vi "practica7MIMO.vi"() -> ()   [LabVIEW 2016]
uses:
  <vilib>/Math Plots/3D Math Plots/3D Mesh/3D Mesh XCtrl/3D Mesh.xctl
  <vilib>/addons/Fuzzy Logic/FL Fuzzy Controller (MIMO).vi
  <vilib>/Math Plots/3D Math Plots/3D Mesh/3D Mesh Datatype/Public/Plot Helper (Matrix).vi
  <vilib>/addons/Fuzzy Logic/NI_Fuzzy_Logic_API.lvlib
  <vilib>/Math Plots/3D Math Plots/3D Mesh/3D Mesh Datatype/3D Mesh Datatype.lvclass
panel:
  out "Waveform Chart 2":dbl[][](graph)
  out "Waveform Chart":dbl[][](graph)
  out "3D Mesh 2":refnum<class "3D Plot Datatype.lvclass">[](xcontrol)
  out "3D Mesh":refnum<class "3D Plot Datatype.lvclass">[](xcontrol)
  out "Motor Derecha":dbl(slide) scale=-100.0..100.0
  out "Motor Izquierda":dbl(slide) scale=-100.0..100.0
  in  "file path":path
  in  "stop":bool
  in  "Reset":bool
  out "Plano de trabajo":picture
  out "Angulo":dbl
  out "Distancia":dbl
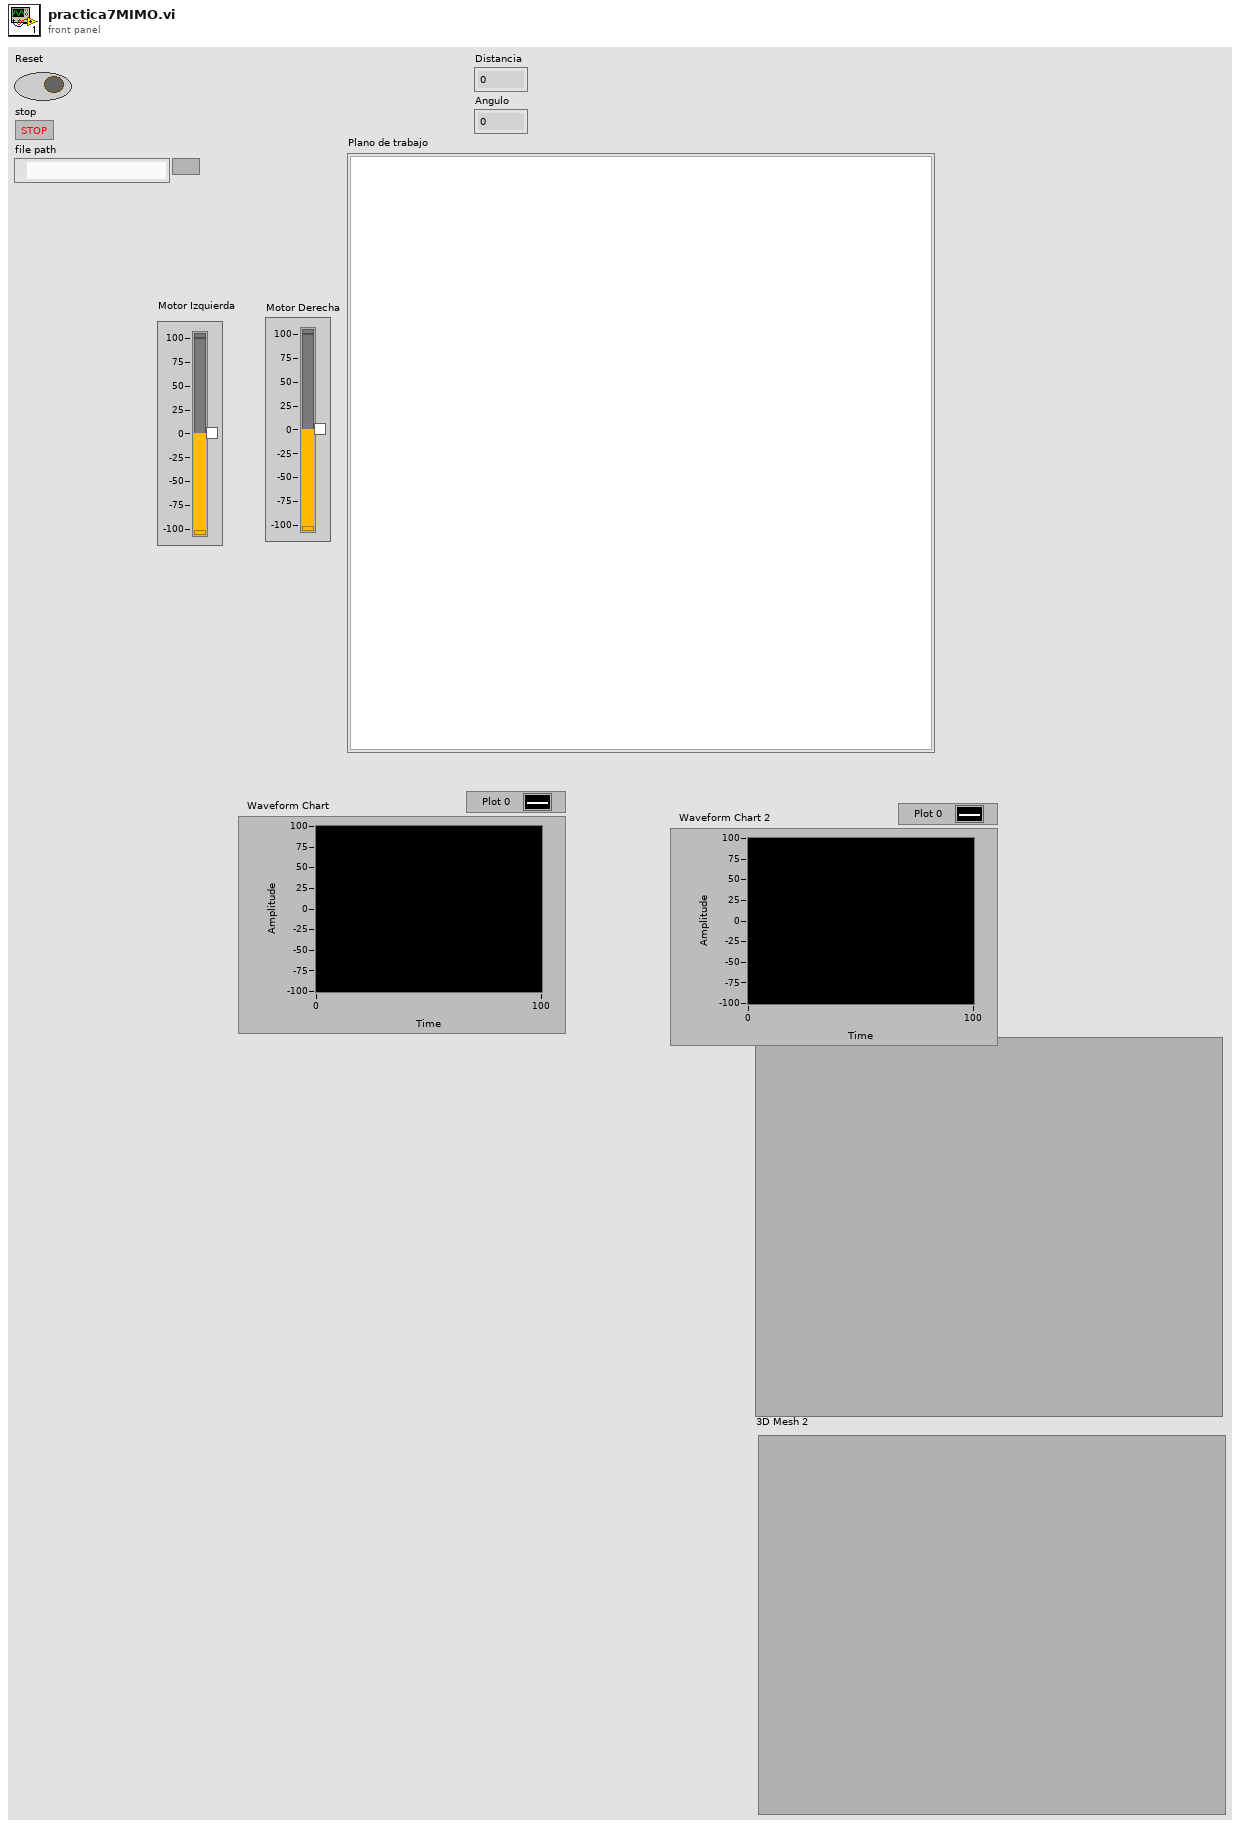
[diagram p1: front panel]
types:
  T1 = typedef "NI_Fuzzy_Logic_API.lvlib/FL System.ctl" = cluster{"input variables":T2[], "output variables":T2[], "rules":T5[], "defuzzification method":T11, "description":string, "user MF interpolating polynomials":T12[]}
  T2 = typedef "NI_Fuzzy_Logic_API.lvlib/FL Variable.ctl" = cluster{"name":string, "range":dbl[], "MFs":T3[]}
  T3 = typedef "NI_Fuzzy_Logic_API.lvlib/FL Membership Function.ctl" = cluster{"name":string, "shape":T4, "points":dbl[], "color":u32, "user-defined shape index":i32}
  T4 = typedef "NI_Fuzzy_Logic_API.lvlib/FL Membership Function Shape.ctl" = u16
  T5 = typedef "NI_Fuzzy_Logic_API.lvlib/FL Rule.ctl" = cluster{"antecedents":T6[], "antecedent connective":T8, "consequents":T9[], "consequent implication":T10, "degree of support":dbl}
  T6 = typedef "NI_Fuzzy_Logic_API.lvlib/FL Antecedent.ctl" = cluster{"Var Index":i32, "MF Index":i32, "Cond":T7}
  T7 = typedef "NI_Fuzzy_Logic_API.lvlib/FL Modifier.ctl" = u16
  T8 = typedef "NI_Fuzzy_Logic_API.lvlib/FL Antecedent Connective.ctl" = u16
  T9 = typedef "NI_Fuzzy_Logic_API.lvlib/FL Consequent.ctl" = cluster{"Var Index":i32, "MF Index":i32, "Cond":T7}
  T10 = typedef "NI_Fuzzy_Logic_API.lvlib/FL Consequent Implication.ctl" = u16
  T11 = typedef "NI_Fuzzy_Logic_API.lvlib/FL Defuzzification.ctl" = u16
  T12 = typedef "NI_Fuzzy_Logic_API.lvlib/FL Interpolating polynomials.ctl" = cluster{"X":dbl[], "Y":dbl[], "Y(x) coeff":dbl[][], "X(y) coeff":dbl[][], "Area(y) coeff":dbl[][], "coa_x(y) coeff":dbl[][]}
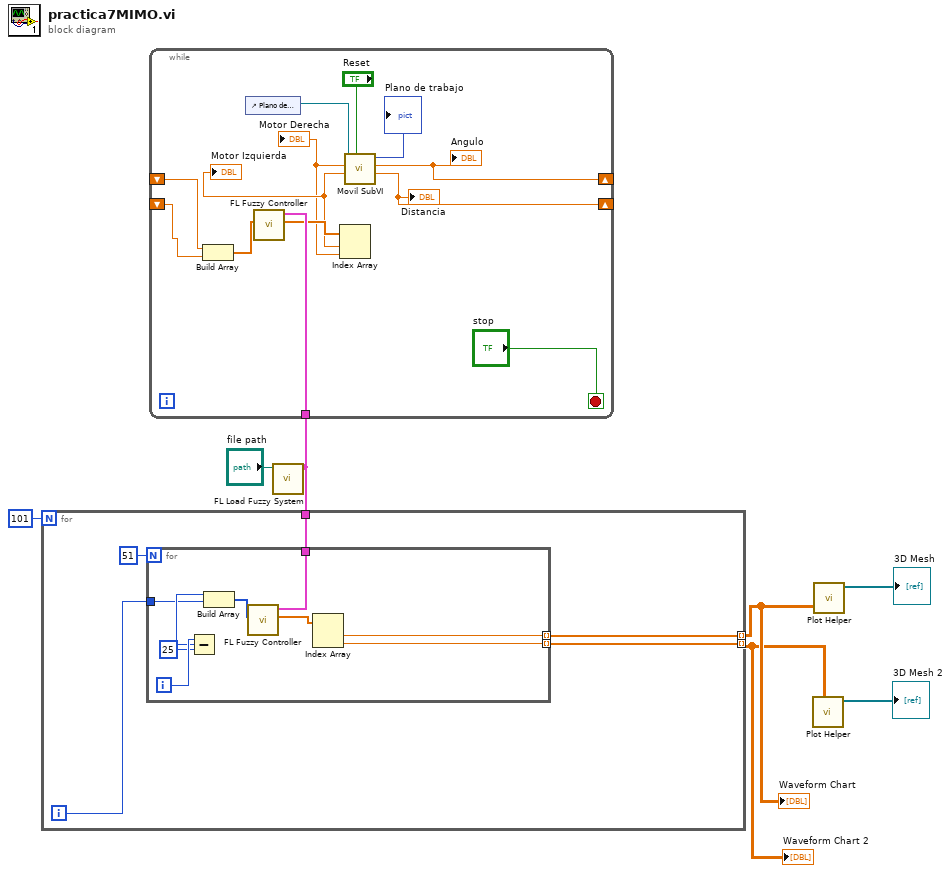
[diagram p0: block diagram]
diagram:
  n1 = call <vilib>:"FL Load Fuzzy System.vi"("file path"="file path") -> ("fuzzy system out"=w5:T1)  [unwired: 9 in, 1 out]
  n2 = for {
    N: 101 -> [_]
    tunnel: [w12] -> w2 mode=indexing
    tunnel: [w11] -> w1 mode=indexing
    tunnel: w5 -> [w8]
    i -> [w9]
    n3 = for {
      N: 51 -> [_]
      tunnel: [w20] -> w12 mode=indexing
      tunnel: [w19] -> w11 mode=indexing
      tunnel: w9 -> [w15]
      tunnel: w8 -> [w13]
      i -> [w18]
      n4 = Subtract(x=w18, y=25) -> (x-y=w16:i32)
      n5 = Build Array(w16, w15) -> (w14:i32[])
      n6 = call-poly <vilib>:"FL Fuzzy Controller.vi"("input values"=w14, "fuzzy system in"=w13) -> ("output values"=w21:dbl[])  [unwired: 5 in, 4 out]
      n7 = Index Array(array=w21) -> (element #1=w20:dbl, element #2=w19:dbl)  [unwired: 2 in]
    }
  }
  "Waveform Chart" <- w2
  "Waveform Chart 2" <- w1
  n8 = while {
    tunnel: w5 -> [w30]
    shift-right: [w28] -> _
    shift-left: _ -> [w25]
    shift-right: [w27] -> _
    shift-left: _ -> [w26]
    stop <- "stop" stop-if-true
    n9 = Build Array(w25, w26) -> (w24:dbl[])
    n10 = control-ref of="Plano de trabajo"() -> (w33:refnum<vi>)
    n11 = call-poly <vilib>:"FL Fuzzy Controller.vi"("input values"=w24, "fuzzy system in"=w30) -> ("output values"=w29:dbl[])  [unwired: 5 in, 4 out]
    n12 = Index Array(array=w29) -> (element #1=w23:dbl, element #2=w22:dbl)  [unwired: 2 in]
    "Motor Izquierda" <- w23
    "Motor Derecha" <- w22
    n13 = call "Movil SubVI.vi"("Reset"="Reset", "Motor Izquierda"=w23, "Motor Derecha"=w22, "Ref Plano"=w33) -> ("Distancia"=w27:dbl, "Angulo"=w28:dbl, "Plano de trabajo"=→"Plano de trabajo":picture)  [unwired: 3 in, 2 out]
    "Distancia" <- w27
    "Angulo" <- w28
  }
  n14 = call-poly <vilib>:"Plot Helper.vi"("z matrix"=w1) -> ("3D Plot lvclass Array out"=→"3D Mesh 2":refnum<class "3D Plot Datatype.lvclass">[])  [unwired: 5 in, 5 out]
  n15 = call-poly <vilib>:"Plot Helper.vi"("z matrix"=w2) -> ("3D Plot lvclass Array out"=→"3D Mesh":refnum<class "3D Plot Datatype.lvclass">[])  [unwired: 5 in, 5 out]
